vi "MWC Get Message.VI"(0 "Timeout ms (-1)":i32) -> (1 "MWC Message Type":T1(ring)=enum."Tune=", 2 "Text":string)   [LabVIEW 2009]
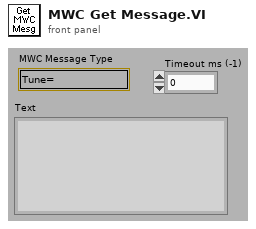
[diagram p1: front panel]
types:
  T1 = enum16{"Bad Message", "No Message", "FMAmplitude=", "FMOffset=", "Tune=", "Switch=", "GenEvent=", "Read", "Ping=", "Stop"}
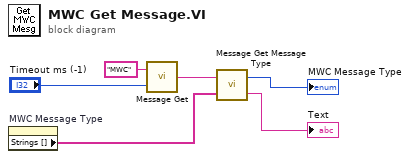
[diagram p0: block diagram]
diagram:
  n1 = property on="MWC Message Type" class="Enum (strict)"() -> ("Strings []"=w1:string[])  [unwired: 2 in, 2 out]
  n2 = call "Message Get.vi"("Timeout ms (-1)"="Timeout ms (-1)", "Module"="MWC") -> ("data out"=w6:string)
  n3 = call "Message Get Message Type.vi"("Message Types"=w1, "Message"=w6) -> ("Trailing text"=→"Text":string, "Message Type"=→"MWC Message Type":i32)
